vi "SetTemperatureSD.vi"(2 "error in (no error)":errorcluster, 3 "temperature":i32) -> (0 "error out":errorcluster, 1 "DLL error code":u32)   [LabVIEW 2015]
doc: "This function will set the desired temperature of the detector. To turn the cooling ON and OFF use the <B>CoolerON</B> and <B>CoolerOFF</B> function respectively.\n\n<B>Parameters:</B>\ntemperature - the temperature in Centigrade.\n Valid range is given by <B>GetTemperatureRange</B>\n\n<B>Error codes:</B>\nDRV_SUCCESS - Accumulations set.\nDRV_NOT_INITIALIZED - System not initialized.\nDRV_ACQUIRING - Acquisition in progress.\nDRV_ERROR_ACK - Unable to communicate with card.\nDRV_P1INVALID - Temperature invalid."
uses:
  DLL/atmcd32d.dll
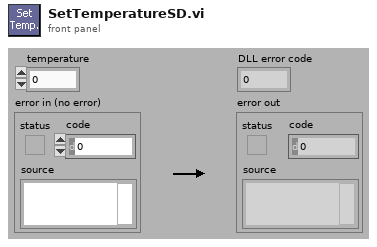
[diagram p1: front panel]
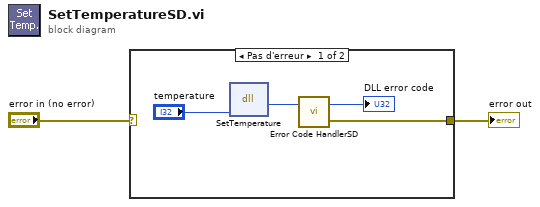
[diagram p0: block diagram]
diagram:
  n1 = case shown="Pas d'erreur" "error in (no error)" {
    selector: "error in (no error)" -> [_ w7]
    tunnel: [w5 w7] -> w1
    frame No Error {
      n2 = dll-call lib="G:/SD/TRANCON-2015/DLL/Atmcd32d.dll" fn="SetTemperature"("temperature"="temperature") -> (w6:u32)  [unwired: 4 in, 2 out]
      n3 = call "Error Code HandlerSD.vi"("DLL error code"=w6) -> ("error out"=w5:errorcluster, "dup DLL error code"=→"DLL error code":u32)  [unwired: 1 in]
    }
    frame Error {
    }
  }
  "error out" <- w1
